vi "Close_Process.vi"(8 "error in (no error)":errorcluster, 11 "Process to kill":string="Winword") -> (0 "error out":errorcluster)   [LabVIEW 2018]
uses:
  psapi.dll
  KERNEL32.DLL
panel:
  out "process handle":u32
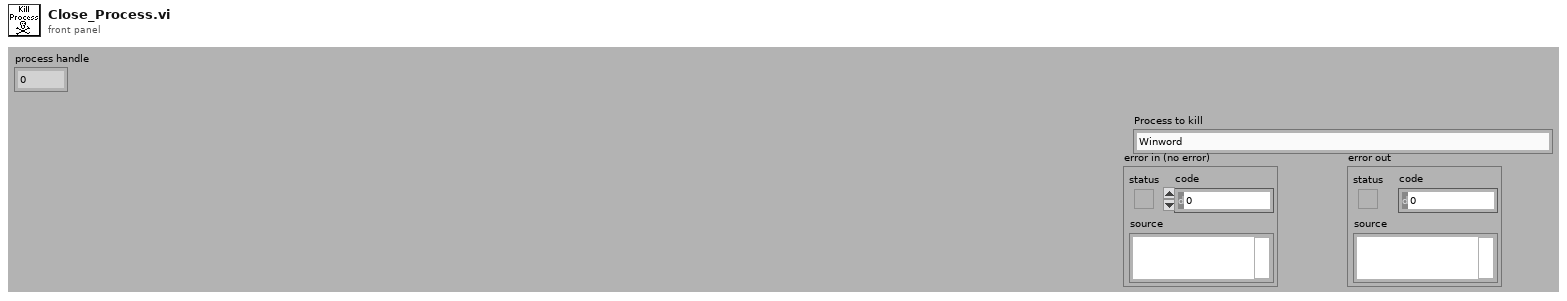
[diagram p1: front panel]
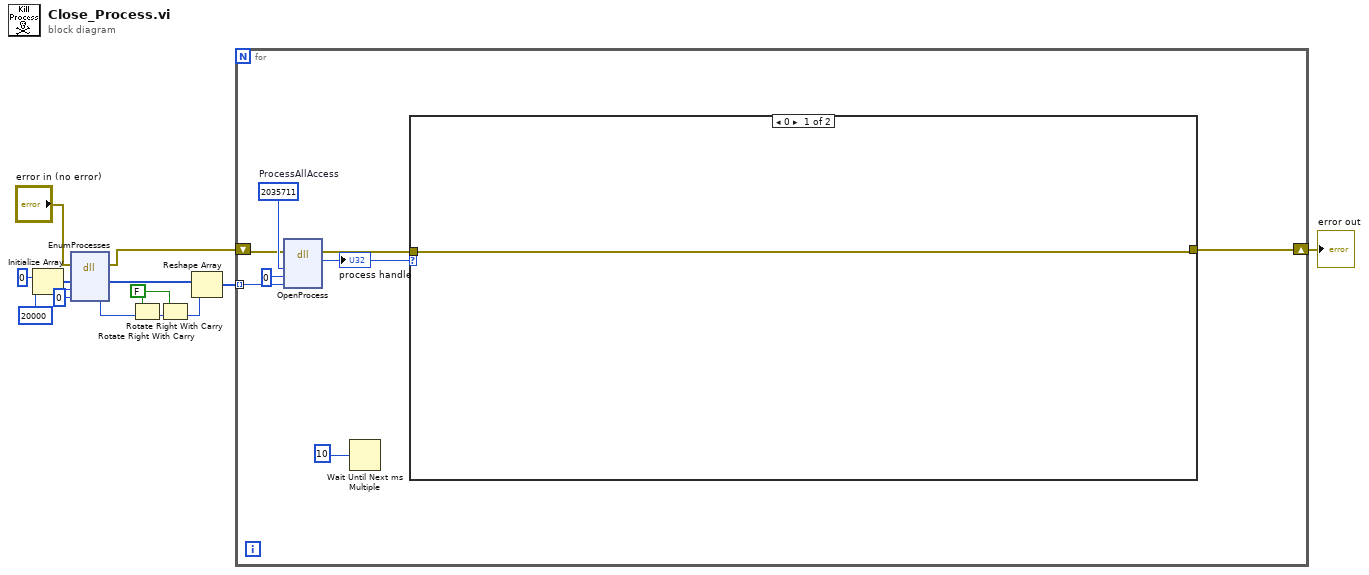
[diagram p0: block diagram]
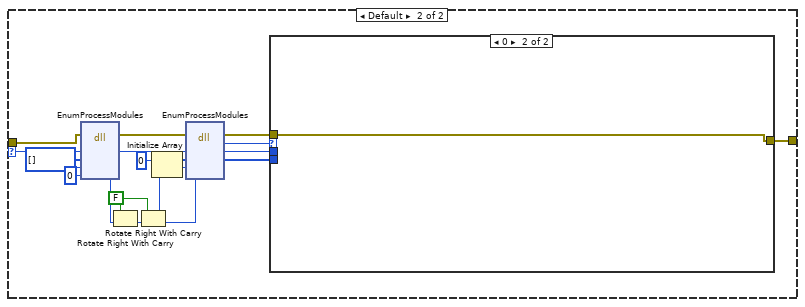
[diagram p2: hidden frame]
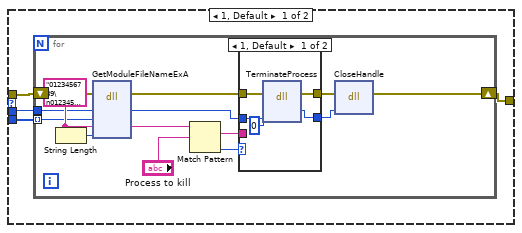
[diagram p3: hidden frame]
diagram:
  w4 = FALSE ("carry")
  w11 = 20000
  n1 = Initialize Array(u32 0, w11) -> (w12:u32[])
  n2 = dll-call lib="psapi.dll" fn="EnumProcesses"(error in="error in (no error)", "lpidProcess"=w12, "cb"=w11, "cbNeeded"=u32 0) -> (error out=w2:errorcluster, "lpidProcess"=w8:u32[], "cbNeeded"=w9:u32)  [unwired: 3 in, 2 out]
  n3 = Rotate Right With Carry(2:w9, 3:w4) -> (0:w6:u32)  [unwired: 1 out]
  n4 = Rotate Right With Carry(2:w6, 3:w4) -> (0:w5:u32)  [unwired: 1 out]
  n5 = Reshape Array(w8, w5) -> (w7:u32[])
  n6 = for {
    tunnel: w7 -> [w19] mode=indexing
    shift-right: [w14] -> w1
    shift-left: w2 -> [w16]
    w17 = 2035711  # ProcessAllAccess
    n7 = dll-call lib="KERNEL32.DLL" fn="OpenProcess"(error in=w16, "dwDesiredAccessas"=w17, "bInheritHandle"=0, "dwProcId"=w19) -> (error out=w15:errorcluster, w18:u32)  [unwired: 5 in, 1 out]
    "process handle" <- w18
    n8 = Wait Until Next ms Multiple(millisecond multiple=10) -> ()  [unwired: 1 out]
    n9 = case shown="0" w18 {
      selector: w18 -> [_ w39]
      tunnel: w15 -> [w22 w26]
      tunnel: [w22 w23] -> w14
      frame 0 {
      }
      frame Default {
        w35 = FALSE ("carry")
        w38 = 0 ("cbNeeded")
        n10 = dll-call lib="psapi.dll" fn="EnumProcessModules"(error in=w26, "hProcesses"=w39, "lphModule"=u32[] [], "cb"=w38, "cbNeeded"=w38) -> (error out=w25:errorcluster, "hProcesses"=w30:u32, "cbNeeded"=w33:i32)  [unwired: 4 in, 2 out]
        n11 = Rotate Right With Carry(2:w33, 3:w35) -> (0:w34:i32)  [unwired: 1 out]
        n12 = Rotate Right With Carry(2:w34, 3:w35) -> (0:w31:i32)  [unwired: 1 out]
        n13 = Initialize Array(u32 0, w31) -> (w32:u32[])
        n14 = dll-call lib="psapi.dll" fn="EnumProcessModules"(error in=w25, "hProcesses"=w30, "lphModule"=w32, "cb"=w31, "cbNeeded"=w31) -> (error out=w24:errorcluster, w29:u32, "hProcesses"=w28:u32, "lphModule"=w27:u32[])  [unwired: 3 in, 2 out]
        n15 = case shown="0" w29 {
          tunnel: w28 -> [w43 _]
          tunnel: w27 -> [w42 _]
          tunnel: w24 -> [w41 w65]
          tunnel: [w40 w65] -> w23
          frame 1, Default {
            n16 = for {
              tunnel: w43 -> [w55]
              tunnel: w42 -> [w54] mode=indexing
              shift-right: [w44] -> w40
              shift-left: w41 -> [w47]
              w56 = "0123456789\n0123456789\n0123456789\n0123456789\n0123456789\n01234567890123456789\n0123456789\n0123456789\n0123456789\n0123456789\n01234567890123456789\n0123456789\n0123456789\n0123456789\n0123456789\n01234567890123456789\n0123456789\n0123456789\n0123456789\n0123456789\n01234567890123456789\n0123456789\n0123456789\n0123456789\n0123456789\n01234567890123456789\n0123456789\n0123456789\n0123456789\n0123456789\n0123456789"
              n17 = String Length(string=w56) -> (length=w57:i32)
              n18 = dll-call lib="psapi.dll" fn="GetModuleFileNameExA"(error in=w47, "hProcess"=w55, "hModule"=w54, "ModuleName"=w56, "nSize"=w57) -> (error out=w46:errorcluster, "hProcess"=w48:u32, "ModuleName"=w50:string)  [unwired: 4 in, 2 out]
              n19 = Match Pattern(string=w50, regular expression="Process to kill") -> (match substring=w49:string, offset past match=w52:i32)  [unwired: 3 out]
              n20 = case shown="1, Default" w52 {
                tunnel: w48 -> [w61 w64]
                tunnel: [w60 w64] -> w51
                tunnel: w49 -> [_ _]
                tunnel: w46 -> [w59 w63]
                tunnel: [w58 w63] -> w45
                frame 1, Default {
                  n21 = dll-call lib="KERNEL32.DLL" fn="TerminateProcess"(error in=w59, "hProcess"=w61, "uExitCode"=0) -> (error out=w58:errorcluster, "hProcess"=w60:u32)  [unwired: 3 in, 2 out]
                }
                frame -1 {
                }
              }
              n22 = dll-call lib="KERNEL32.DLL" fn="CloseHandle"(error in=w45, "Handle"=w51) -> (error out=w44:errorcluster)  [unwired: 3 in, 2 out]
            }
          }
          frame 0 {
          }
        }
      }
    }
  }
  "error out" <- w1
